vi "REC_Query RATE.vi"(0 "System no.":i32=1 min=1 max=4 step=1, 2 "RecorderIDs to query":string[](array[string]), 5 "error in":errorcluster) -> (14 "Reording rate":i32[](array[numeric]), 19 "error out":errorcluster)   [LabVIEW 2020]
doc: "REC? RATE (Get Recording Rate)\n\nDescription \nQueries the recording rate for the data recorders of the controller.\n\nFormat\nREC? RATE[ <RecorderID>]\n\nArguments\nREC? RATE without arguments queries all data recorders of the controller.\n<RecorderID>\nData recorder, whose configuration is to be queried; to be specified as alias (p. 94) \nThe available data recorders can be queried with USG? SYS (p. 80). \nPossible values: REC_1 to RECn, where n = number of data recorders in the controller\nResponse\n{<RecorderID> = <RecordingRate> LF}\nSee REC RATE (p. 35) for further details.\nExample\n>> REC? RATE\n<< REC_1 = 1\n<< REC_2 = 1\n\nNotes\nFor further details, see \"Data Recorder - GCS 3.0\" (p. 107). \n\nUser command level\nUSR"
panel:
  # "REC? RATE (Get Recording Rate)\n\nQueries the recording rate for the data recorders of the controller."
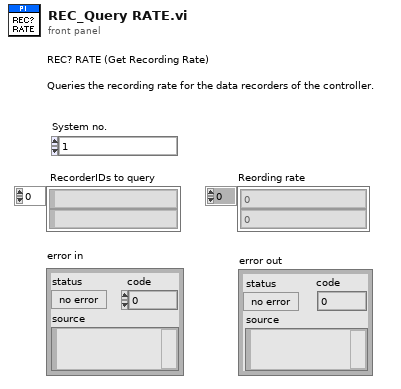
[diagram p1: front panel]
types:
  T1 = typedef "Syntax.ctl" = enum16{"GCS 1.0", "GCS 2.0", "GCS 3.0"}
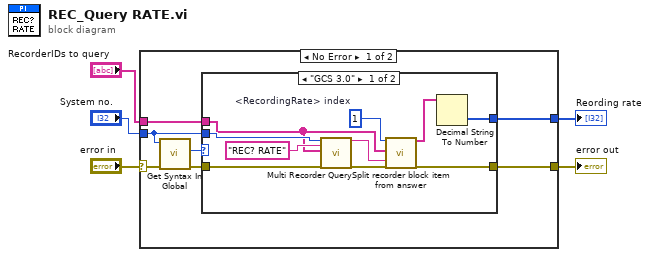
[diagram p0: block diagram]
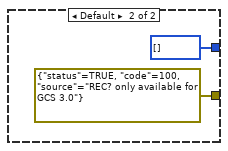
[diagram p2: hidden frame]
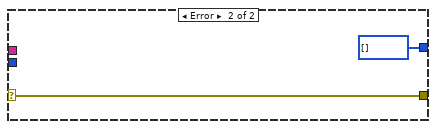
[diagram p3: hidden frame]
diagram:
  n1 = case shown="No Error" "error in" {
    selector: "error in" -> [w12 w26]
    tunnel: [w9 w26] -> w2
    tunnel: "RecorderIDs to query" -> [w7 _]
    tunnel: "System no." -> [w6 _]
    tunnel: [w8 i32[] [] ("Number of recorded data points")] -> w1
    frame No Error {
      n2 = call "Get Syntax In Global.vi"("error in"=w12, "System no."=w6) -> ("error out"=w10:errorcluster, "Syntax"=w11:T1)  [unwired: 8 in]
      n3 = case shown="\"GCS 3.0\"" w11 {
        tunnel: w10 -> [w20 _]
        tunnel: [w13 errorcluster {"status"=TRUE, "code"=100, "source"="REC? only available for GCS 3.0"} ("error out")] -> w9
        tunnel: [w17 i32[] [] ("Number of recorded data points")] -> w8
        tunnel: w7 -> [w16 _]
        tunnel: w6 -> [w22 _]
        frame "GCS 3.0" {
          w19 = 1  # <RecordingRate> index
          n4 = call "Multi Recorder Query.vi"("System no."=w22, "Recorder Command"="REC? RATE" ("format string"), "RecorderIDs to query"=w16, "error in"=w20) -> ("Answer"=w15:string, "error out"=w14:errorcluster)  [unwired: 14 in]
          n5 = call "Split recorder block item from answer.vi"("Slice block item"=w19, "RecorderIDs to query"=w16, "Input string"=w15, "error in"=w14) -> ("Sliced text segments"=w18:string[], "error out"=w13:errorcluster)  [unwired: 14 in]
          n6 = Decimal String To Number(string=w18) -> (number=w17:i32[])  [unwired: 2 in, 1 out]
        }
        frame Default {
        }
      }
    }
    frame Error {
    }
  }
  "error out" <- w2
  "Reording rate" <- w1
